vi "Lookup Nodes.vi"(8 "error in (no error)":errorcluster, 11 "Sequencing Control in":refnum<class "Sequencing Control.lvclass">) -> (0 "error out":errorcluster, 3 "Sequencing Control out":refnum<class "Sequencing Control.lvclass">)   [LabVIEW 2020, in "VolatusSeqGUI.lvlib" / "Sequencing Control.lvclass"]
uses:
  Sequencing Control.lvclass
  Sequencing Control.lvclass/Sequencing Control.ctl
  Volatus/VolatusAPI/VolatusAPI.lvclass
  VolatusConfig/VolatusConfigElement/VolatusConfigElement.lvclass
  VolatusConfig/VolatusConfig.lvlib
  VolatusConfig/Meta Type.ctl
  VolatusConfig/Meta Name.ctl
  lv-cdm/CDM-Config/Config Element/Config Element.lvclass
  Sequencing Task.ctl
  VolatusConfig/Node/Node Config.lvclass
  C:/dev/lv20CE/relink/lv-volatus/VolatusConfig/VolatusConfigElement/VolatusConfigElement.lvclass
  C:/dev/lv20CE/relink/lv-volatus/VolatusConfig/Node/Node Config.lvclass
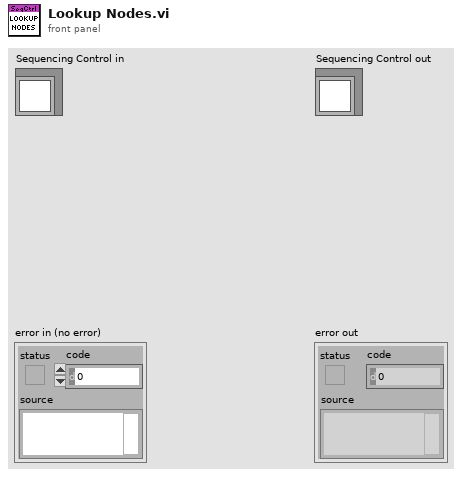
[diagram p1: front panel]
types:
  T1 = typedef "VolatusSeqGUI.lvlib/Sequencing Control.lvclass/Sequencing Task.ctl" = cluster{"Node":string, "Task":string}
  T2 = typedef "VolatusConfig.lvlib/Meta Name.ctl" = enum16{"VL_Type", "VL_Node_IP", "VL_Node_Type", "VL_Task_Type", "VL_Group_Type", "VL_Channel_Type", "VL_Channel_DataType", "VL_Config_Version", "VL_Overlay_Type", "VL_Config_Hash"}
  T3 = typedef "VolatusConfig.lvlib/Meta Type.ctl" = enum16{"UNKNOWN", "VL_System", "VL_Cluster", "VL_Node", "VL_Task", "VL_Group", "VL_Channel", "VL_Task_List", "VL_Scaling", "VL_Sensor", "VL_Sensor_List", "VL_Scale"}
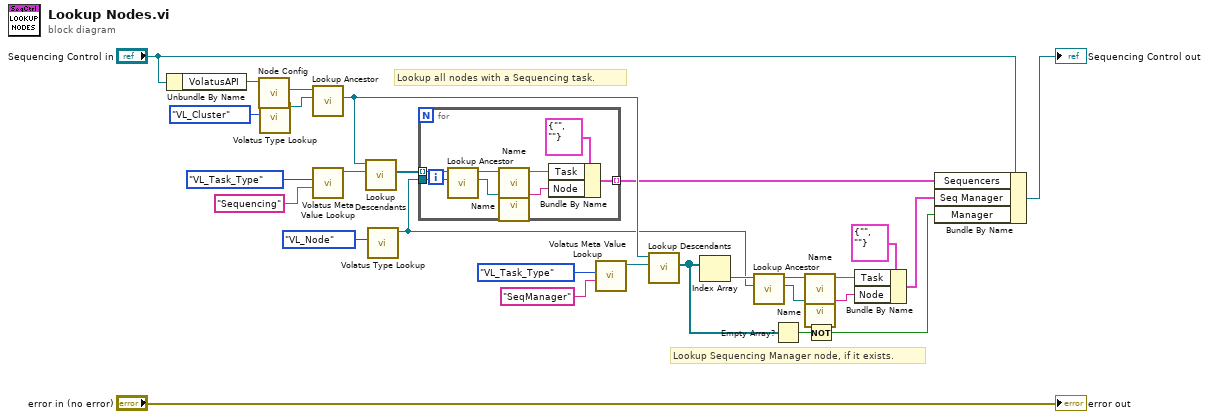
[diagram p0: block diagram]
diagram:
  # "Lookup Sequencing Manager node, if it exists."
  # "Lookup all nodes with a Sequencing task."
  n1 = Unbundle By Name("Sequencing Control in") -> ("VolatusAPI"=w1:refnum<class "VolatusAPI.lvclass">)
  n2 = call "Node Config.vi"("VolatusAPI in"=w1) -> ("Node Config"=w27:refnum<class "Node Config.lvclass">)  [unwired: 9 in, 1 out]
  n3 = call "Volatus Type Lookup.vi"("Meta Type"=Meta_Type."VL_Cluster") -> ("Config Lookup out"=w25:refnum<class "Config Lookup.lvclass">)  [unwired: 9 in, 1 out]
  n4 = call "Lookup Ancestor.vi"("Lookup"=w25, "VolatusConfigElement in"=w27) -> ("Ancestor"=w16:refnum<class "Config Element.lvclass">)  [unwired: 7 in, 2 out]
  n5 = call "Volatus Meta Value Lookup.vi"("Value"="Sequencing", "Meta Name"=Meta_Name."VL_Task_Type") -> ("Config Lookup out"=w22:refnum<class "Config Lookup.lvclass">)  [unwired: 8 in, 1 out]
  n6 = call "Lookup Descendants.vi"("Lookup"=w22, "Config Element in"=w16) -> ("Descendants"=w21:refnum<class "Config Element.lvclass">[])  [unwired: 7 in, 2 out]
  n7 = call "Volatus Type Lookup.vi"("Meta Type"=Meta_Type."VL_Node") -> ("Config Lookup out"=w7:refnum<class "Config Lookup.lvclass">)  [unwired: 9 in, 1 out]
  n8 = for {
    tunnel: w21 -> [w36] mode=indexing
    tunnel: w7 -> [w35]
    tunnel: [w29] -> w3 mode=indexing
    n9 = call "Lookup Ancestor.vi"("Lookup"=w35, "Config Element in"=w36) -> ("Ancestor"=w33:refnum<class "Config Element.lvclass">, "Config Element out"=w34:refnum<class "Config Element.lvclass">)  [unwired: 7 in, 1 out]
    n10 = call "Name.vi"("Config Element in"=w34) -> ("Name"=w31:string)  [unwired: 9 in, 1 out]
    n11 = call "Name.vi"("Config Element in"=w33) -> ("Name"=w30:string)  [unwired: 9 in, 1 out]
    n12 = Bundle By Name(cluster=T1 {"Node"="", "Task"=""} ("Sequencing Task"), "Task"=w31, "Node"=w30) -> (w29:T1)
  }
  n13 = call "Volatus Meta Value Lookup.vi"("Value"="SeqManager", "Meta Name"=Meta_Name."VL_Task_Type") -> ("Config Lookup out"=w19:refnum<class "Config Lookup.lvclass">)  [unwired: 8 in, 1 out]
  n14 = call "Lookup Descendants.vi"("Lookup"=w19, "Config Element in"=w16) -> ("Descendants"=w9:refnum<class "Config Element.lvclass">[])  [unwired: 7 in, 2 out]
  n15 = Index Array(array=w9) -> (element=w10:refnum<class "Config Element.lvclass">)  [unwired: 1 in]
  n16 = call "Lookup Ancestor.vi"("Lookup"=w7, "Config Element in"=w10) -> ("Ancestor"=w12:refnum<class "Config Element.lvclass">, "Config Element out"=w11:refnum<class "Config Element.lvclass">)  [unwired: 7 in, 1 out]
  n17 = Empty Array?(array=w9) -> (empty?=w8:bool)
  n18 = call "Name.vi"("Config Element in"=w11) -> ("Name"=w14:string)  [unwired: 9 in, 1 out]
  n19 = call "Name.vi"("Config Element in"=w12) -> ("Name"=w15:string)  [unwired: 9 in, 1 out]
  n20 = Not(x=w8) -> (.not. x?=w5:bool)
  n21 = Bundle By Name(cluster=T1 {"Node"="", "Task"=""} ("Sequencing Task"), "Task"=w14, "Node"=w15) -> (w4:T1)
  n22 = Bundle By Name(cluster="Sequencing Control in", "Sequencers"=w3, "Seq Manager"=w4, "Manager"=w5) -> (→"Sequencing Control out":refnum<class "Sequencing Control.lvclass">)
  "error out" <- "error in (no error)"
